vi "Initialize Logger Instance.vi"(8 "error in (no error)":errorcluster, 11 "Logger Reference":refnum<data-value>) -> (0 "error out":errorcluster, 3 "LoggerReference out":refnum<class "LoggerReference.lvclass">)   [LabVIEW 2017, in "Composed Log.lvlib" / "LoggerReference.lvclass"]
uses:
  LoggerReference.lvclass
  Types/MessageCluster.ctl
  LoggerReference.lvclass/LoggerReference.ctl
  Composed Log.lvlib
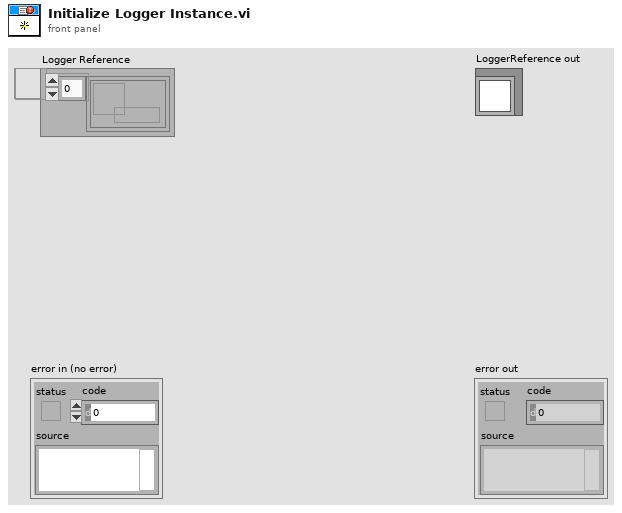
[diagram p1: front panel]
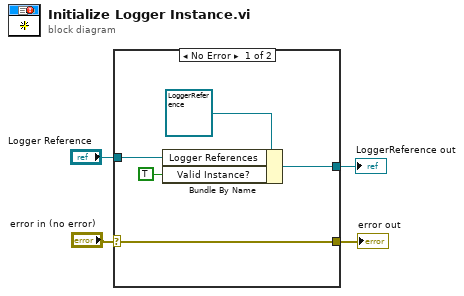
[diagram p0: block diagram]
diagram:
  n1 = case shown="No Error" "error in (no error)" {
    selector: "error in (no error)" -> [w5 w10]
    tunnel: "Logger Reference" -> [w8 _]
    tunnel: [w7 _] -> w3
    tunnel: [w5 w10] -> w1
    frame No Error {
      n2 = Bundle By Name(cluster=refnum<class "LoggerReference.lvclass"> refnum ("Composed Log.lvlib:LoggerReference.lvclass"), "Logger References"=w8, "Valid Instance?"=TRUE) -> (w7:refnum<class "LoggerReference.lvclass">)
    }
    frame Error {
    }
  }
  "error out" <- w1
  "LoggerReference out" <- w3
